vi "Soft Stops.vi"(0 "Motor In":dbl=0.04, 1 "Disable Softstops":bool, 2 "Disable Motor":bool, 3 "correlation":bool=TRUE, 5 "Sense":dbl, 9 "Lo Limit":dbl=-10.0, 11 "Hi Limit":dbl=35.0, 12 "Speed near Limit":dbl=0.02, 13 "Margin":dbl=1.0, 14 "Motor Coerce":dbl=1.0) -> (4 "Motor Out":dbl, 10 "At Lo":bool, 15 "At Hi":bool)   [LabVIEW 2012]
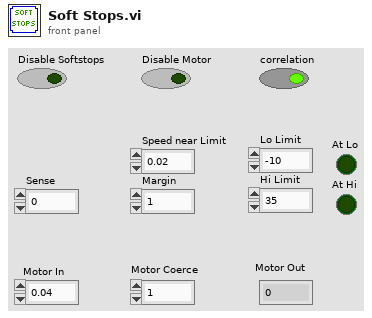
[diagram p1: front panel]
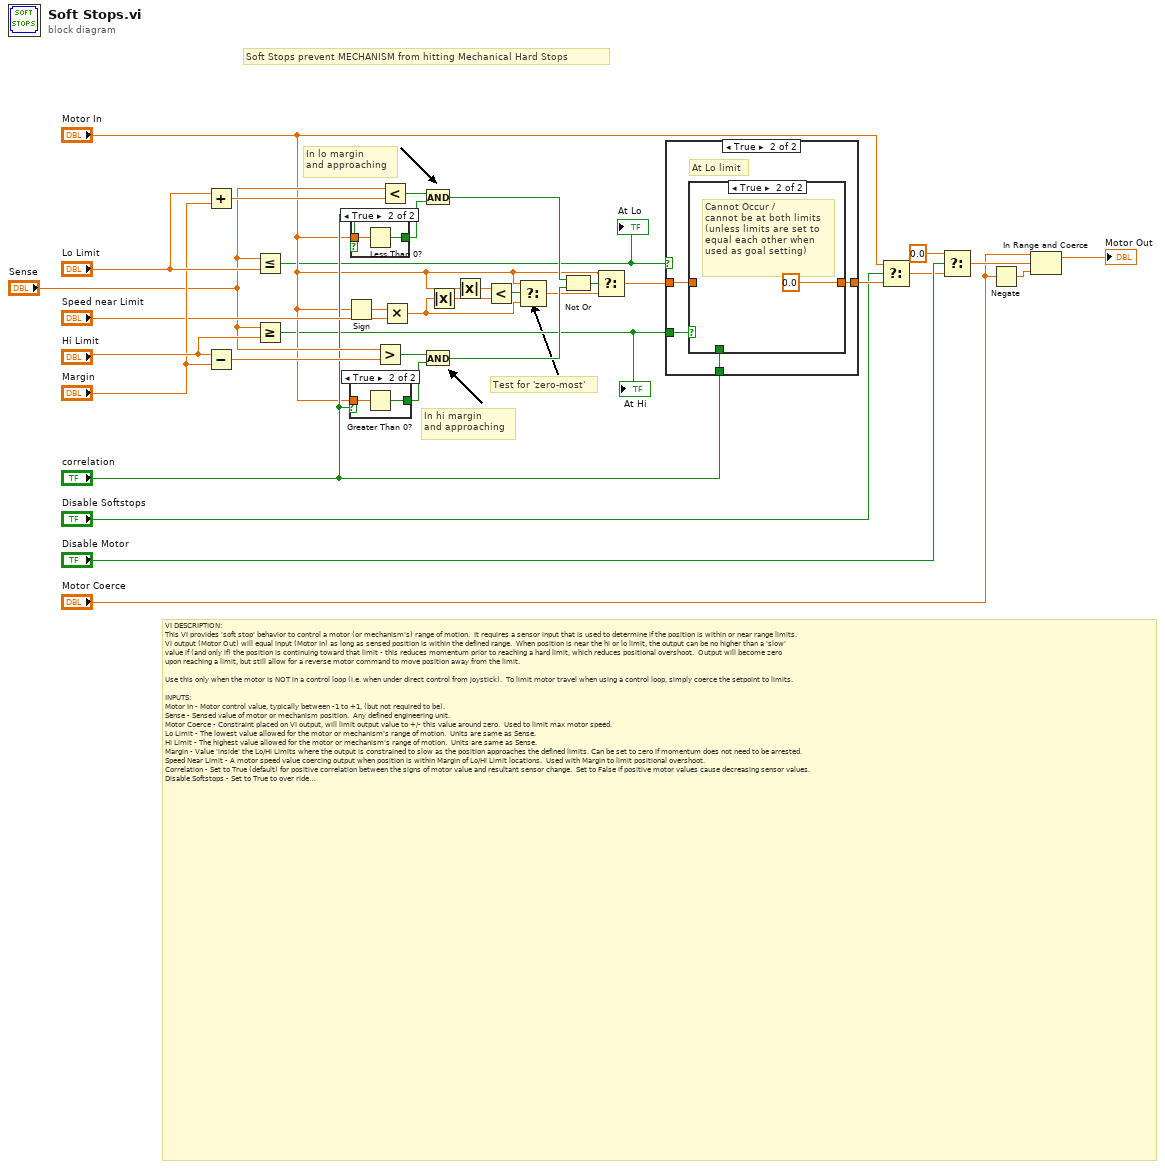
[diagram p0: block diagram]
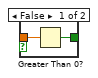
[diagram p2: hidden frame]
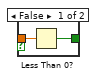
[diagram p3: hidden frame]
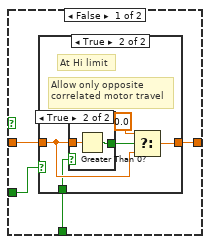
[diagram p4: hidden frame]
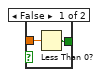
[diagram p6: hidden frame]
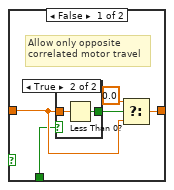
[diagram p7: hidden frame]
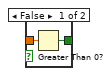
[diagram p8: hidden frame]
diagram:
  # "In hi margin\nand approaching"
  # "In lo margin\nand approaching"
  # "Test for 'zero-most'"
  # "VI DESCRIPTION:\nThis VI provides 'soft stop' behavior to control a motor (or mechanism's) range of motion.  It requires a sensor input that is used to determine if the position is within or near range limits.\nVI output (Motor Out) will equal input (Motor In) as long as sensed position is within the defined range.  When position is near the hi or lo limit, the output can be no higher than a 'slow'\nvalue if (and only if) the position is continuing toward that limit - this reduces momentum prior to reaching a hard limit, which reduces positional overshoot.  Output will become zero \nupon reaching a limit, but still allow for a reverse motor command to move position away from the limit.\n\nUse this only when the motor is NOT in a control loop (i.e. when under direct control from joystick).  To limit motor travel when using a control loop, simply coerce the setpoint to limits.\n\nINPUTS:\nMotor In - Motor control value, typically between -1 to +1, (but not required to be).\nSense - Sensed value of motor or mechanism position.  Any defined engineering unit.\nMotor Coerce - Constraint placed on VI output, will limit output value to +/- this value around zero.  Used to limit max motor speed.\nLo Limit - The lowest value allowed for the motor or mechanism's range of motion.  Units are same as Sense.\nHi Limit - The highest value allowed for the motor or mechanism's range of motion.  Units are same as Sense.\nMargin - Value 'inside' the Lo/Hi Limits where the output is constrained to slow as the position approaches the defined limits. Can be set to zero if momentum does not need to be arrested.\nSpeed Near Limit - A motor speed value coercing output when position is within Margin of Lo/Hi Limit locations.  Used with Margin to limit positional overshoot.\nCorrelation - Set to True (default) for positive correlation between the signs of motor value and resultant sensor change.  Set to False if positive motor values cause decreasing sensor values.\nDisable Softstops - Set to True to over ride the softstop behavor and pass Motor In directly to Motor Out.\nDisable Motor - Set to True to send value zero to Motor Output.  If both Disables are selected, Disable Motor takes precedence over Disable Softstops.\n\nOUTPUTS:\nMotor Out - Motor control value modified by VI behavior.\nAt Lo - Boolean indicating status of sensed position, True if equal or lower than Lo Limit.\nAt Hi - Boolean indicating status of sensed position, True if equal or higher than Hi Limit.\n\nIMPLEMENTATION:\nDo not use in a control loop, instead use setpoint coercion for this situation.  For direct motor control:\nDetermine the correlation of the mechanical arrangement; if positive motor values cause increasing sensor values, set Correlation to True.\nDetermine the physical limits of the mechanism and set Lo and Hi Limits just short of these limits, by an amount that will accomodate any small overshoot that might remain after tuning.\nTo limit positional overshoot, create a region just inside each limit to slow the motor by setting Margin.\nSet Speed Near Limit to a value slow enough to bring the mechanism to a stop prior to reaching physical limits.\nSet Motor Coerce to the maximum speed that the mechanism is allowed to travel.\nExperimentally determine values that minimize the Margin region and maximize Speed Near Limit, without striking the mechanism's physical limits when approaching at full speed.\n\n\nFIRST Team 836, RoboBees"
  # "Soft Stops prevent MECHANISM from hitting Mechanical Hard Stops"
  n1 = Add(x="Lo Limit", y="Margin") -> (x+y=w18:dbl)
  n2 = Subtract(x="Hi Limit", y="Margin") -> (x-y=w14:dbl)
  n3 = Less Or Equal?(x="Sense", y="Lo Limit") -> (x <= y?=w2:bool)
  "At Lo" <- w2
  n4 = Greater Or Equal?(x="Sense", y="Hi Limit") -> (x >= y?=w1:bool)
  "At Hi" <- w1
  n5 = Sign(1:"Motor In") -> (0:w22:dbl)
  n6 = case shown="True" "correlation" {
    tunnel: [w35 w37] -> w13
    tunnel: "Motor In" -> [w36 w38]
    frame False {
      n7 = Less Than 0?(x=w36) -> (x < 0?=w35:bool)
    }
    frame True {
      n8 = Greater Than 0?(x=w38) -> (x > 0?=w37:bool)
    }
  }
  n9 = case shown="True" "correlation" {
    tunnel: [w40 w42] -> w17
    tunnel: "Motor In" -> [w39 w41]
    frame False {
      n10 = Greater Than 0?(x=w39) -> (x > 0?=w40:bool)
    }
    frame True {
      n11 = Less Than 0?(x=w41) -> (x < 0?=w42:bool)
    }
  }
  n12 = Greater?(x="Sense", y=w14) -> (0:w16:bool)
  n13 = Less?(x="Sense", y=w18) -> (x < y?=w19:bool)
  n14 = Multiply(x=w22, y="Speed near Limit") -> (x*y=w4:dbl)
  n15 = And(x=w19, y=w17) -> (x .and. y?=w12:bool)
  n16 = And(x=w16, y=w13) -> (x .and. y?=w11:bool)
  n17 = Absolute Value(x=w4) -> (abs(x)=w6:dbl)
  n18 = Absolute Value(x="Motor In") -> (abs(x)=w7:dbl)
  n19 = Less?(x=w7, y=w6) -> (x < y?=w8:bool)
  n20 = Select(t="Motor In", s=w8, f=w4) -> (s? t:f=w5:dbl)
  n21 = Not Or(1:w11, 2:w12) -> (0:w10:bool)
  n22 = Select(t="Motor In", s=w10, f=w5) -> (s? t:f=w20:dbl)
  n23 = case shown="True" w2 {
    tunnel: [w45 w59] -> w33
    tunnel: w20 -> [w46 w60]
    tunnel: "correlation" -> [w44 w58]
    tunnel: w1 -> [w43 w57]
    frame False {
      n24 = case shown="True" w43 {
        tunnel: w46 -> [w47 w50]
        tunnel: [w47 w49] -> w45
        tunnel: w44 -> [_ w48]
        frame False {
          # "At neither limit"
        }
        frame True {
          # "Allow only opposite\ncorrelated motor travel"
          # "At Hi limit"
          n25 = case shown="True" w48 {
            tunnel: [w54 w55] -> w52
            tunnel: w50 -> [w53 w56]
            frame False {
              n26 = Less Than 0?(x=w53) -> (x < 0?=w54:bool)
            }
            frame True {
              n27 = Greater Than 0?(x=w56) -> (x > 0?=w55:bool)
            }
          }
          n28 = Select(t=0.0, s=w52, f=w50) -> (s? t:f=w49:dbl)
        }
      }
    }
    frame True {
      # "At Lo limit"
      n29 = case shown="True" w57 {
        tunnel: w60 -> [w62 _]
        tunnel: [w63 0.0 ("Turret Yaw Control")] -> w59
        tunnel: w58 -> [w61 _]
        frame False {
          # "Allow only opposite\ncorrelated motor travel"
          n30 = case shown="True" w61 {
            tunnel: [w67 w68] -> w65
            tunnel: w62 -> [w66 w69]
            frame False {
              n31 = Greater Than 0?(x=w66) -> (x > 0?=w67:bool)
            }
            frame True {
              n32 = Less Than 0?(x=w69) -> (x < 0?=w68:bool)
            }
          }
          n33 = Select(t=0.0, s=w65, f=w62) -> (s? t:f=w63:dbl)
        }
        frame True {
          # "Cannot Occur / \ncannot be at both limits\n(unless limits are set to\nequal each other when\nused as goal setting)"
        }
      }
    }
  }
  n34 = Select(t="Motor In", s="Disable Softstops", f=w33) -> (s? t:f=w26:dbl)
  n35 = Select(t=0.0, s="Disable Motor", f=w26) -> (s? t:f=w32:dbl)
  n36 = Negate(x="Motor Coerce") -> (-x=w31:dbl)
  n37 = In Range and Coerce(upper limit="Motor Coerce", x=w32, lower limit=w31) -> (coerced(x)=→"Motor Out":dbl)  [unwired: 1 out]
